vi "Test.vi"(10 "w":dbl, 11 "v":dbl) -> (2 "Vr":dbl, 3 "Vl":dbl)   [LabVIEW 2017]
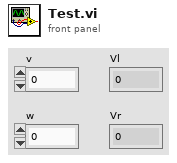
[diagram p1: front panel]
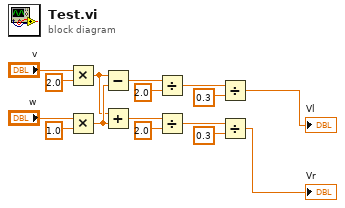
[diagram p0: block diagram]
diagram:
  n1 = Multiply(x="v", y=2.0) -> (x*y=w9:dbl)
  n2 = Multiply(x="w", y=1.0) -> (x*y=w10:dbl)
  n3 = Subtract(x=w9, y=w10) -> (x-y=w14:dbl)
  n4 = Add(x=w9, y=w10) -> (x+y=w6:dbl)
  n5 = Divide(x=w14, y=2.0) -> (x/y=w12:dbl)
  n6 = Divide(x=w6, y=2.0) -> (x/y=w7:dbl)
  n7 = Divide(x=w12, y=0.3) -> (x/y=→"Vl":dbl)
  n8 = Divide(x=w7, y=0.3) -> (x/y=→"Vr":dbl)
